vi "QUERY_TELEM_all_temp.vi"(8 "error in":errorcluster, 11 "TRXmode":u16(ring)=1 items=["QUERY_TELEM_2 (V)"=2, "QUERY_TELEM_1 (H)"=1]) -> (0 "error out":errorcluster, 3 "Temp_8pcs":i32[](array[numeric]), 4 "all_data":i32[](array[numeric]))   [LabVIEW 2023, in "Clover_Cell.lvlib"]
uses:
  Clover_Cell.lvlib
panel:
  in  "TCPIPin":T1={"address"="192.168.100.111", "remote port or service name"=5025, "timeout ms (60000)"=10000}
  # "CLC_Gen4_L2"
  # "AiP_1 : 0\nAiP_2 : 1\nAiP_3 : 2\nAiP_4 : 3\nAiP_5 : 4\nAiP_6 : 5\nAiP_7 : 6\nAiP_8 : 7"
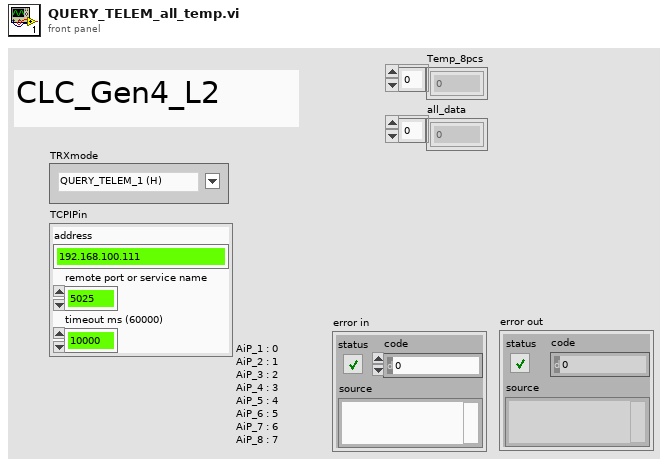
[diagram p1: front panel]
types:
  T1 = cluster{"address":string, "remote port or service name":u16, "timeout ms (60000)":i32}
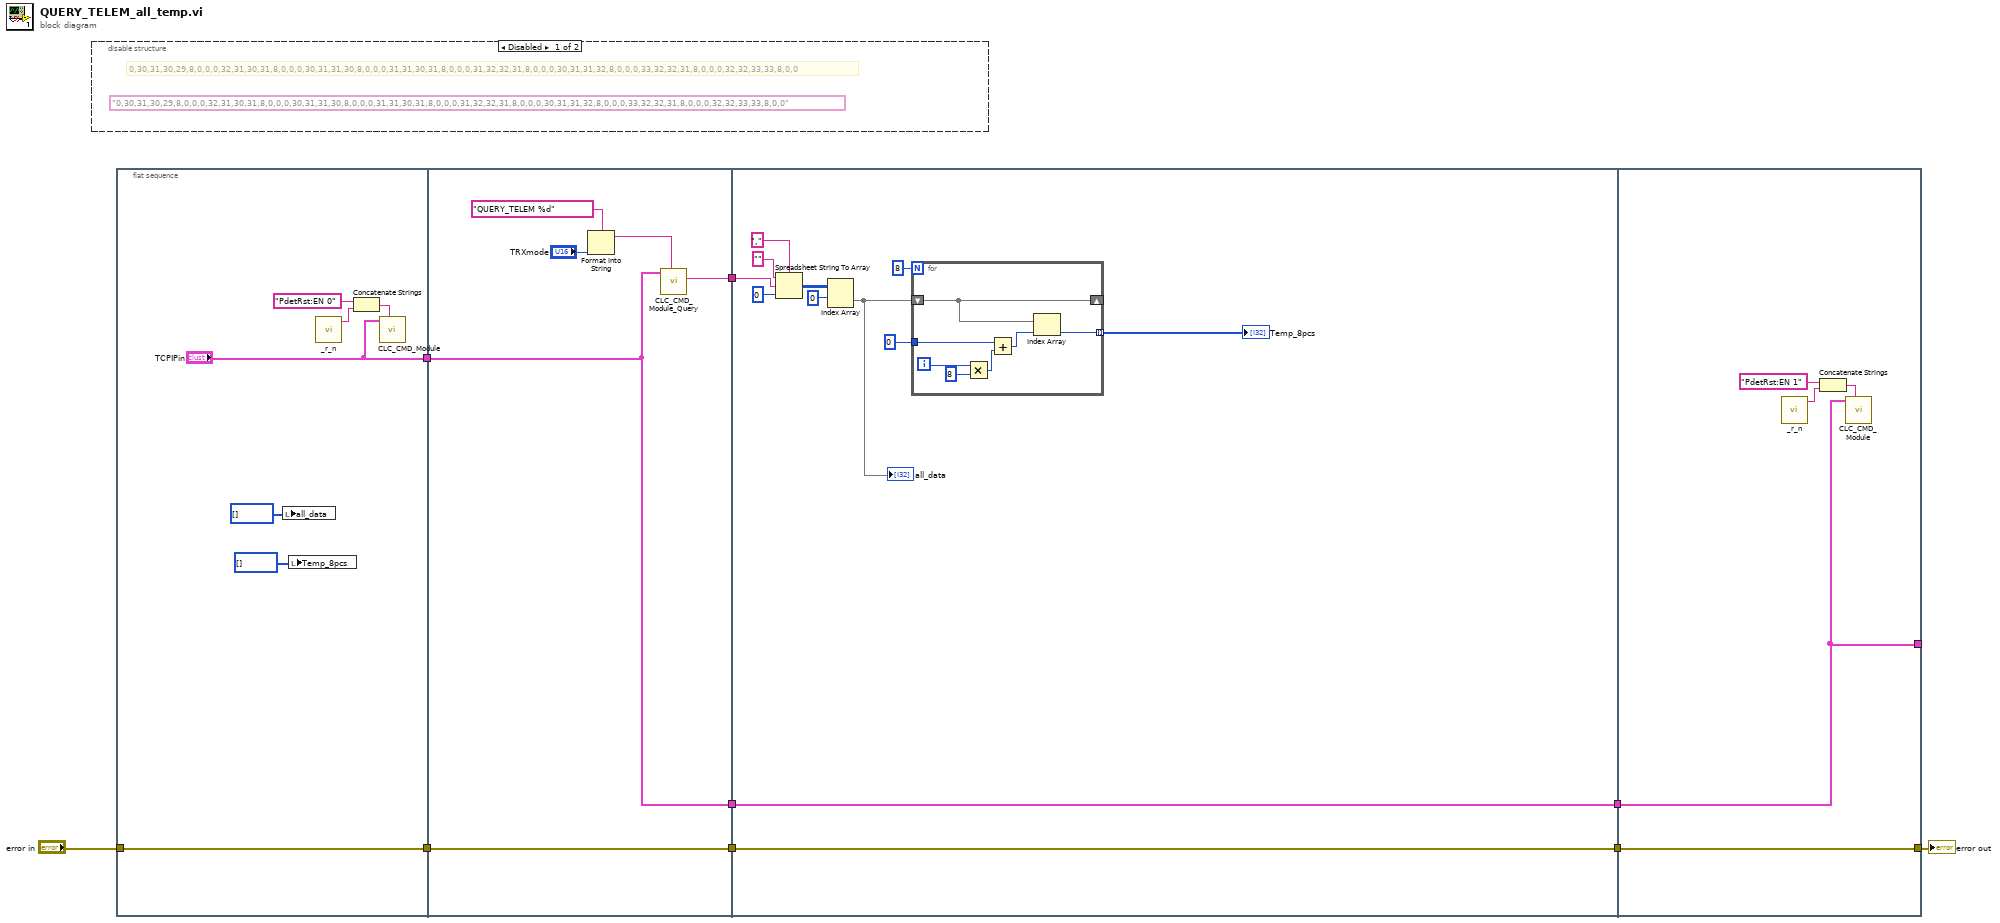
[diagram p0: block diagram]
diagram:
  n1 = disable-structure shown="Disabled" {
    frame Disabled {
      (unwired) "0,30,31,30,29,8,0,0,0,32,31,30,31,8,0,0,0,30,31,31,30,8,0,0,0,31,31,30,31,8,0,0,0,31,32,32,31,8,0,0,0,30,31,31,32,8,0,0,0,33,32,32,31,8,0,0,0,32,32,33,33,8,0,0"
      # "0,30,31,30,29,8,0,0,0,32,31,30,31,8,0,0,0,30,31,31,30,8,0,0,0,31,31,30,31,8,0,0,0,31,32,32,31,8,0,0,0,30,31,31,32,8,0,0,0,33,32,32,31,8,0,0,0,32,32,33,33,8,0,0"
    }
    frame Enabled {
    }
  }
  n2 = flat-sequence {
    tunnel: ["TCPIPin"] -> w7
    tunnel: "error in" -> [w12]
    tunnel: [w12] -> w2
    tunnel: [w22] -> w9
    tunnel: [w18] -> w8
    tunnel: w7 -> [w18]
    tunnel: [w17] -> w3
    tunnel: w2 -> [w17]
    tunnel: w9 -> [w32]
    tunnel: w8 -> [w28]
    tunnel: [w28] -> w6
    tunnel: [w27] -> w4
    tunnel: w3 -> [w27]
    tunnel: [w43] -> _
    tunnel: w6 -> [w43]
    tunnel: [w42] -> w1
    tunnel: w4 -> [w42]
    frame #0 {
      n3 = local write "all_data"(i32[] [] ("all_data")) -> ()
      n4 = local write "Temp_8pcs"(i32[] [] ("Temp_8pcs")) -> ()
      n5 = call "_r_n.vi"() -> ("command"=w15:string)  [unwired: 5 in]
      n6 = Concatenate Strings("PdetRst:EN 0" ("CMD in"), w15) -> (w14:string)
      n7 = call "CLC_CMD_Module.vi"("CMD in"=w14, "TCPIPin"="TCPIPin") -> ()  [unwired: 6 in, 4 out]
    }
    frame #1 {
      n8 = Format Into String(format string="QUERY_TELEM %d" ("data in"), "TRXmode") -> (resulting string=w19:string)  [unwired: 2 in, 1 out]
      n9 = call "CLC_CMD_Module_Query.vi"("CMD in"=w19, "TCPIPin"=w18) -> ("data out"=w22:string)  [unwired: 7 in, 2 out]
    }
    frame #2 {
      n10 = Spreadsheet String To Array(delimiter (Tab)=",", format string="", spreadsheet string=w32, array type (2D Dbl)=0) -> (array=w29:i32[][])
      n11 = Index Array(array=w29, index (row)=0 ("disabled index (col)")) -> (element=w24:i32[])  [unwired: 1 in]
      "all_data" <- w24
      n12 = for {
        N: 8 -> [_]
        tunnel: 0 ("disabled index (col)") -> [w38]
        shift-right: [w41] -> _
        shift-left: w24 -> [w41]
        tunnel: [w35] -> w23 mode=indexing
        i -> [w40]
        n13 = Multiply(x=w40, y=8) -> (x*y=w37:i32)
        n14 = Add(x=w38, y=w37) -> (x+y=w36:i32)
        n15 = Index Array(array=w41, index=w36) -> (element=w35:i32)
      }
      "Temp_8pcs" <- w23
    }
    frame #3 {
      n16 = call "_r_n.vi"() -> ("command"=w45:string)  [unwired: 5 in]
      n17 = Concatenate Strings("PdetRst:EN 1" ("CMD in"), w45) -> (w46:string)
      n18 = call "CLC_CMD_Module.vi"("CMD in"=w46, "TCPIPin"=w43) -> ()  [unwired: 6 in, 4 out]
    }
  }
  "error out" <- w1
